vi "Meas Check Sequence Files.vi"(8 "error in":errorcluster, 11 "sequence setup":T1) -> (0 "error out":errorcluster, 2 "cancel?":bool, 3 "sequence setup out (copy)":T1)   [LabVIEW 2013]
doc: "This VI will check if there are some files with filenames that collides with file name base of the new measurement. If so, it will as operator to either remove them or cancel."
uses:
  Meas Sequence Configuration.ctl
  Meas Sampling Configuration.ctl
  adc/ADC Trig Config.ctl
  adc/ADC Trig Mode Source.ctl
  adc/ADC Trig Coupling.ctl
  adc/ADC Trig Slope.ctl
  processing/QWTB/Meas Proc QWTB Algorithm Parameter Data.ctl
  Meas Range Mode.ctl
  Meas Sampling Rate Mode.ctl
  varilib/varilib.lvlib
panel:
  in  "btn cancel":bool
  in  "btn rem":bool
  out "Files to remove":string
  # "Following existing files collides with the new measurement file names.\nDo you want to REMOVE them or CANCEL the operation and change file names?"
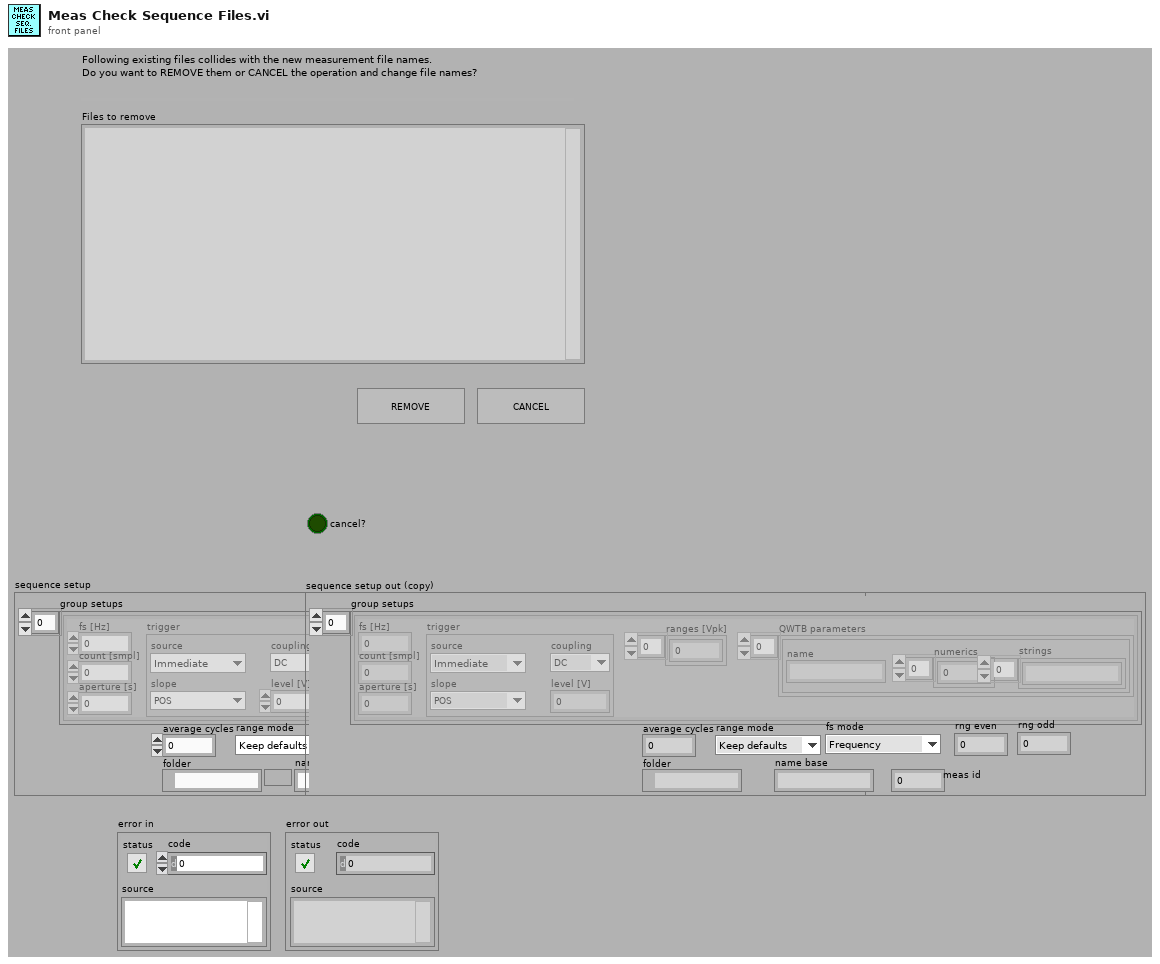
[diagram p1: front panel]
types:
  T1 = typedef "Meas Sequence Configuration.ctl" = cluster{"group setups":T2[], "average cycles":i32, "range mode":T8, "fs mode":T9, "rng even":dbl, "rng odd":dbl, "folder":path, "name base":string, "meas id":i32}
  T2 = typedef "Meas Sampling Configuration.ctl" = cluster{"fs [Hz]":dbl, "count [smpl]":i64, "aperture [s]":dbl, "trigger":T3, "ranges [Vpk]":dbl[], "QWTB parameters":T7[]}
  T3 = typedef "ADC Trig Config.ctl" = cluster{"source":T4, "level [V]":dbl, "coupling":T5, "slope":T6}
  T4 = typedef "ADC Trig Mode Source.ctl" = enum16{"Immediate", "External", "Level"}
  T5 = typedef "ADC Trig Coupling.ctl" = enum16{"DC", "AC"}
  T6 = typedef "ADC Trig Slope.ctl" = enum16{"POS", "NEG"}
  T7 = typedef "Meas Proc QWTB Algorithm Parameter Data.ctl" = cluster{"name":string, "numerics":dbl[], "strings":string[]}
  T8 = typedef "Meas Range Mode.ctl" = enum16{"Keep defaults", "Set All channels", "Set Odd and Even channels"}
  T9 = typedef "Meas Sampling Rate Mode.ctl" = enum16{"Frequency", "Period"}
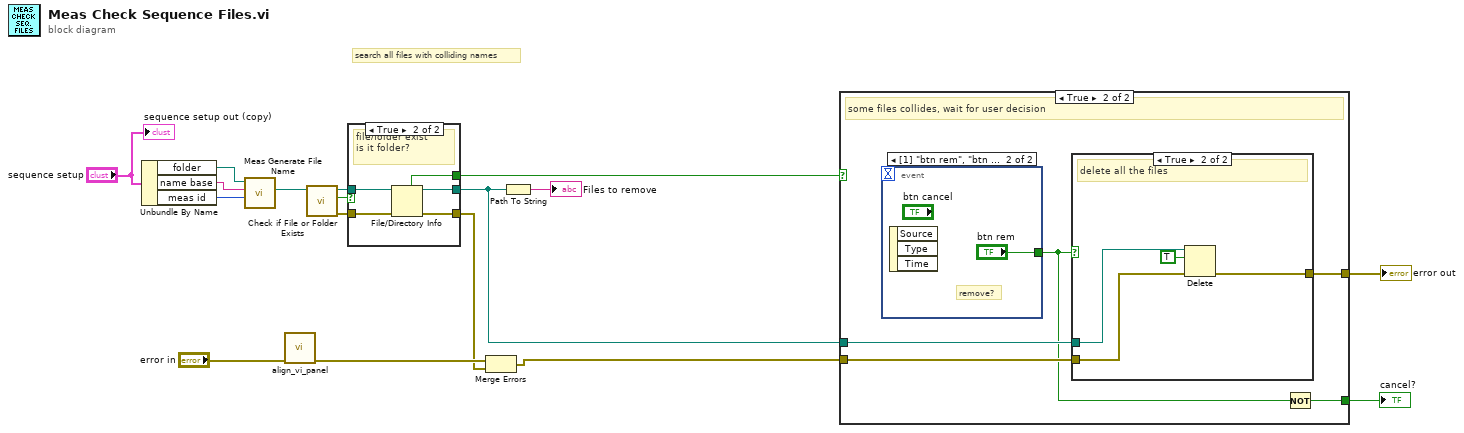
[diagram p0: block diagram]
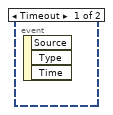
[diagram p5: hidden frame]
diagram:
  # "search all files with colliding names"
  n1 = Unbundle By Name("sequence setup") -> ("folder"=w13:path, "name base"=w12:string, "meas id"=w11:i32)
  n2 = call "Meas Generate File Name.vi"("meas id"=w11, "name base"=w12, "folder"=w13) -> ("measurement root folder"=w10:path)  [unwired: 4 in, 4 out]
  n3 = call "align_vi_panel.vi"("error in"="error in") -> ("error out"=w6:errorcluster)  [unwired: 10 in]
  n4 = call <vilib>:"Check if File or Folder Exists.vi"("path"=w10) -> ("error out"=w8:errorcluster, "file or folder exists?"=w7:bool, "dup path"=w9:path)  [unwired: 8 in]
  n5 = case shown="True" w7 {
    tunnel: w9 -> [w18 w24]
    tunnel: w8 -> [w19 w23]
    tunnel: [_ w22] -> w3
    tunnel: [w19 w21] -> w5
    tunnel: [w18 w20] -> w1
    frame False {
    }
    frame True {
      # "file/folder exist\nis it folder?"
      n6 = File/Directory Info(path=w24, error in=w23) -> (path out=w20:path, directory=w22:bool, error out=w21:errorcluster)  [unwired: 4 out]
    }
  }
  n7 = Merge Errors(w6, w5) -> (w2:errorcluster)
  n8 = Path To String(path=w1) -> (string=→"Files to remove":string)
  n9 = case shown="True" w3 {
    tunnel: w1 -> [_ w30]
    tunnel: w2 -> [w25 w29]
    tunnel: [w25 w28] -> w16
    tunnel: [_ w27] -> w15
    frame False {
      # "no files collides, go away"
    }
    frame True {
      # "some files collides, wait for user decision"
      n10 = event shown="[1] \"btn rem\", \"btn cancel\": Value Change;  Panel Close" {
        selector: _ -> [_ _]
        dyn-events: _ -> [_ _]
        timeout: _ -> [_ _]
        tunnel: [_ "btn rem"] -> w26
        event Timeout {
          n11 = event-data() -> ()  [unwired: 1 in, 3 out]
        }
        event "btn rem", "btn cancel": Value Change; Panel Close {
          # "remove?"
          n12 = event-data() -> ()  [unwired: 1 in, 3 out]
        }
      }
      n13 = case shown="True" w26 {
        tunnel: w30 -> [_ w35]
        tunnel: w29 -> [w31 w34]
        tunnel: [w31 w33] -> w28
        frame False {
        }
        frame True {
          # "delete all the files"
          n14 = Delete(path (use dialog)=w35, entire hierarchy (F)=TRUE, error in=w34) -> (error out=w33:errorcluster)  [unwired: 2 in, 2 out]
        }
      }
      n15 = Not(x=w26) -> (.not. x?=w27:bool)
    }
  }
  "error out" <- w16
  "cancel?" <- w15
  "sequence setup out (copy)" <- "sequence setup"
